vi "Alpha Ver 1.1.vi"() -> ()   [LabVIEW 2015]
uses:
  <instrlib>/Keithley 622x LV 2009/Configure/Source/Typedefs/KE622x -- Current Range.ctl
  <instrlib>/Keithley 622x LV 2009/Configure/Source/Typedefs/KE622x -- Current Ranges.ctl
  <instrlib>/Keithley 622x LV 2009/Typedefs/KE622x -- On Off Control.ctl
  <instrlib>/Keithley 622x LV 2009/Utility/Typedefs/KE622x -- Instrument Type.ctl
  <instrlib>/Keithley 622x LV 2009/Configure/Source/Typedefs/KE622x -- Voltage Limit.ctl
  <instrlib>/Keithley 2000/Public/Configure/Configure DC Volts.vi
  <userlib>/LV-Link3/PolySubVIs/DtCreateAinChan.vi
  <userlib>/LV-Link3/PolySubVIs/DtOLReadMultipleSingle.vi
  <instrlib>/Keithley 2000/Keithley 2000.lvlib
  <instrlib>/Keithley 622x LV 2009/Keithley 622x.lvlib
panel:
  out "DAQ A4":dbl format="%#_13g"
  out "DAQ_clust":T1
  out "DAQ A3":dbl format="%#_13g"
  out "DAQ A2":dbl format="%#_13g"
  out "DAQ A1":dbl format="%#_13g"
  out "Real stop cur":dbl format="%#_13g"
  out "Real start cur":dbl format="%#_13g"
  in  "Stop cur prefix":u16(ring)=2
  in  "Start cur prefix":u16(ring)=2
  out "MULTIPLE GRAPHS":cluster{dbl[], dbl[]}[](graph)
  in  "X-Axis":T2(ring)
  in  "Range":u8(ring)=20 items=["100nV", "200nV", "500nV", "1µV", "2µV", "5µV", "10µV", "20µV", "50µV", "100µV", "200µV", "500µV", "1mV", "2mV", "5mV", "10mV", "20mV", "50mV", "100mV", "200mV", "500mV", "1V"]
  in  "Display Type copy":u16(ring)=3 items=["X %", "Y %", "X Calibrated", "Y Calibrated", "Mag %", "Mag Calibrated", "Phase Degrees", "Ratio", "ADC 1", "ADC 2", "ADC 3", "ADC 4 ", "Noise %", "Noise Calibrated", "Ref Frequency", "", ""]
  out "Units copy":string
  out "Display copy":dbl format="%.3f"
  out "Overload":bool
  out "Display":dbl format="%.3f"
  out "Units":string
  in  "Display Type":u16(ring)=2 items=["X %", "Y %", "X Calibrated", "Y Calibrated", "Mag %", "Mag Calibrated", "Phase Degrees", "Ratio", "ADC 1", "ADC 2", "ADC 3", "ADC 4 ", "Noise %", "Noise Calibrated", "Ref Frequency", "", ""]
  in  "Time Constant":u16(ring) items=["MIN", "1ms", "3ms", "10ms", "30ms", "100ms", "300ms", "1s", "3s", "10s", "30s", "100s", "300s"]
  in  "Slope":u8(ring) items=["6db/octave", "12dB/octave"]
  in  "Dynamic Reserve":u16(ring) items=["High Stability", "Normal", "High Reserve"]
  in  "Auto Sensitivity":bool
  in  "Auto Measure":bool
  out "6221_error_out":errorcluster
  out "2000_error_out":errorcluster
  out "5110_error_out":errorcluster
  out "Input Mode":i32(ring) items=[" Voltage Input (A or A-B) ", "Current Input 10E6 V/A", "Current Input 10E8 V/A"]
  out "5110":refnum<visa-resource-name>
  in  "GPIB Address":i8=11 min=1 max=32 step=1
  out "DAQ A0":dbl format="%#_13g"
  out "2000":dbl format="%#_13g"
  in  "Device":string(combo)
  in  "Number \nof points":i32
  in  "Folder\nprename":string
  out "TIME GRAPH":cluster{dbl[], dbl[]}[](graph)
  out "T0":u32
  out "LIMIT":bool
  out "LIMIT":bool
  out "Error Code":string
  in  "Comments":string
  out "file":refnum<file>
  out "2000":refnum<visa-resource-name>
  out "6221":refnum<visa-resource-name>
  out "Step  (A)":dbl=5e-05 format="%#_3p"
  in  "Stop\ncurrent (A)":dbl=2.0 format="%#_6p"
  in  "Start \ncurrent (A)":dbl=1.0 format="%#_6p"
  in  "Check For SCPI Errors? (T)":bool=TRUE
  out "Interlock Tripped?":bool
  out "Compliance?":bool
  in  "Turn Off Output \nIf Compliance?":bool=TRUE
  in  "Turning ON/OFF\ncurrent output":T3=enum."On"
  in  "Range Selection":T4={"Auto Range?"=TRUE, "Man / Selected\nRange"=enum."2nA"}
  # "FILE CONFIGURATION"
  # "ADMIN PANEL"
  # "KEITHLEY 6221 CONFIGURATION (ADMIN ONLY)"
  # "KEITHLEY DAQ CONFIGURATION (ADMIN ONLY)"
  # "PRINCETON LOCK-IN AMP (ADMIN ONLY)"
  # "I don't know what the hell it is,\njust don't touch it"
  # "SENSITIVITY"
  # "INPUT CONFIGURATION"
  # "READINGS"
  # "START, STOP, STEP, CONFIGURATION"
  # "IF ON"
  # "Output Channels Time - Constant \nSlope & Dynamic Reserve"
  # "Compliance = Limiting output voltage\nThis switch determines if we want to switch \noff the current output if wee exceed compliance"
  # "LOCK-IN READINGS"
  # "RIGHT DISPLAY"
  # "LEFT DISPLAY"
  # "There is a safe switch at \nthe back of the instrument \nThis indicator shows if it is on"
  # "You have hit a damn jackpot \nby exceeding the limited voltage\nCongrats"
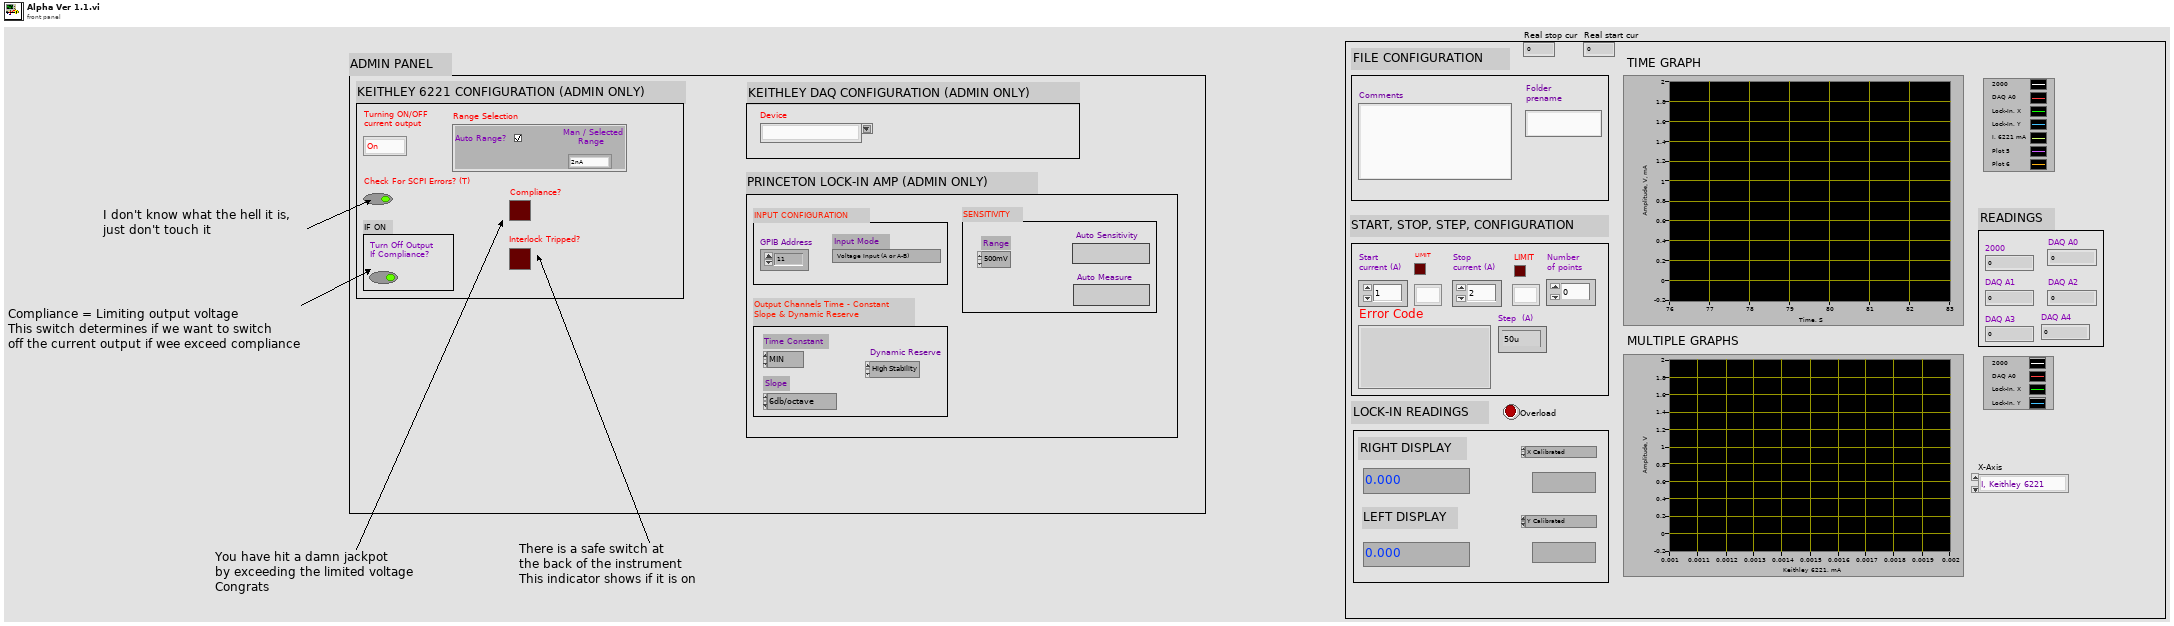
[diagram p1: front panel]
types:
  T1 = cluster{"Task out":i32, "Actual Number of Channels":u32, "error out":errorcluster}
  T2 = enum16{"I, Keithley 6221", "V, Keithley 2000", "V, Keithley DAQ A0", "V, Keithley DAQ A1", "V, Keithley DAQ A2", "V, Keithley DAQ A3", "V, Lock-In X", "V, Lock-In Y"}
  T3 = typedef "Keithley 622x.lvlib/KE622x -- On Off Control.ctl" = enum16{"Off", "On"}
  T4 = typedef "Keithley 622x.lvlib/KE622x -- Current Range.ctl" = cluster{"Auto Range?":bool, "Man / Selected\nRange":T5}
  T5 = typedef "Keithley 622x.lvlib/KE622x -- Current Ranges.ctl" = enum16{"2nA", "20nA", "200nA", "2uA", "20uA", "200uA", "2mA", "20mA", "100mA"}
  T6 = typedef "Keithley 622x.lvlib/KE622x -- Instrument Type.ctl" = enum16{"KE6220", "KE6221"}
  T7 = typedef "Keithley 622x.lvlib/KE622x -- Voltage Limit.ctl" = dbl
  T8 = cluster{"Task out":i32, "error out":errorcluster}
  T9 = cluster{dbl[], dbl[], dbl[], dbl[], dbl[], dbl[], dbl[], dbl[], dbl[]}
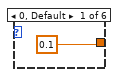
[diagram p2: hidden frame]
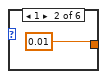
[diagram p3: hidden frame]
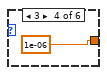
[diagram p4: hidden frame]
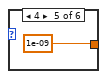
[diagram p5: hidden frame]
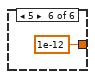
[diagram p6: hidden frame]
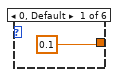
[diagram p7: hidden frame]
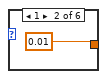
[diagram p8: hidden frame]
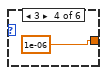
[diagram p9: hidden frame]
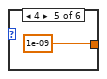
[diagram p10: hidden frame]
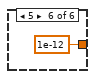
[diagram p11: hidden frame]
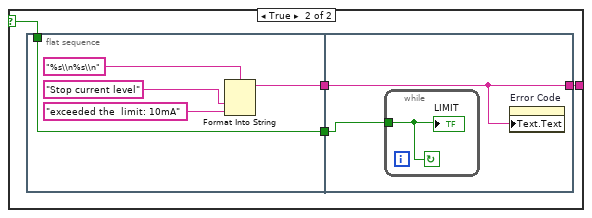
[diagram p12: hidden frame]
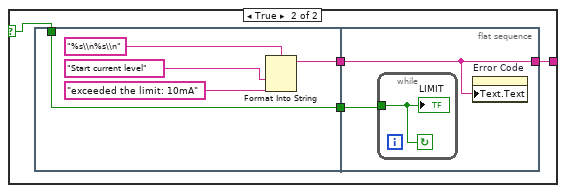
[diagram p13: hidden frame]
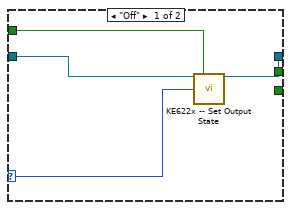
[diagram p14: hidden frame]
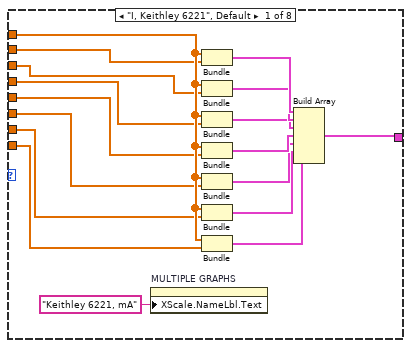
[diagram p15: hidden frame]
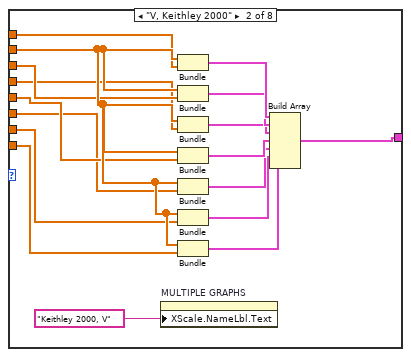
[diagram p16: hidden frame]
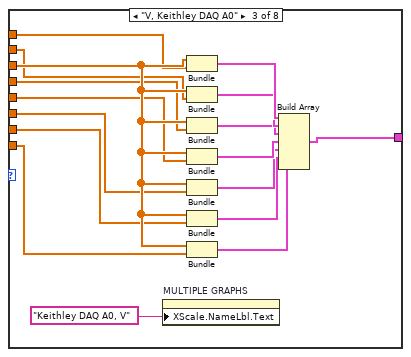
[diagram p17: hidden frame]
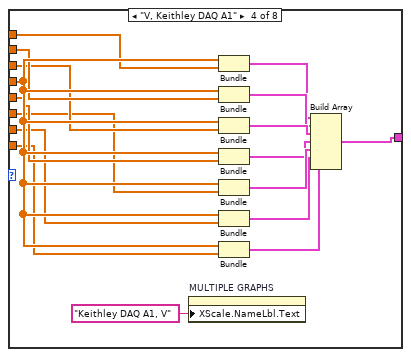
[diagram p18: hidden frame]
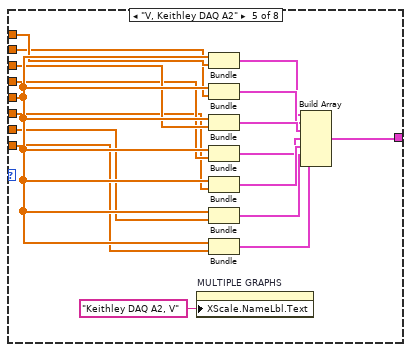
[diagram p19: hidden frame]
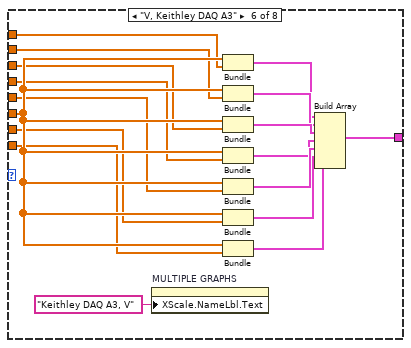
[diagram p20: hidden frame]
diagram:
  n1 = flat-sequence {
    tunnel: [w173] -> w7
    tunnel: [w172] -> w6
    tunnel: [w171] -> w5
    tunnel: [w170] -> w4
    tunnel: [w169] -> w3
    tunnel: [w168] -> w2
    tunnel: [w157] -> w1
    tunnel: w7 -> [w755]
    tunnel: w6 -> [w754]
    tunnel: w5 -> [w753]
    tunnel: w4 -> [w752]
    tunnel: w3 -> [w751]
    tunnel: w2 -> [w750]
    tunnel: w1 -> [w749]
    frame #0 {
      # "File configuration"
      # "Start, Stop, Step"
      # "Time Intit"
      # "Initializing instruments"
      n2 = flat-sequence {
        frame #0 {
          w16 = TRUE  # reset
          w15 = FALSE  # ID query
          # "Initialize Lock-In 5110"
          # "Initialize Keithley 2000"
          # "Initialize Keithley 6221"
          n3 = call <instrlib>:"Initialize.vi"("VISA resource name"=refnum<visa-resource-name> "KEITHLEY_MULTIMETER") -> ("VISA resource name out"=w20:refnum<visa-resource-name>)  [unwired: 17 in, 1 out]
          n4 = call <instrlib>:"Initialize.vi"("VISA resource name"=refnum<visa-resource-name> "KEITHLEY_DC_AC_CURRENT_SOURCE", "Error Queue Option"=enum16{"Clear Error Queue", "Error Query"}."Clear Error Queue", "Instrument Type"=KE622x_--_Instrument_Type."KE6221") -> ("VISA resource name out"=→"6221":refnum<visa-resource-name>, "error out"=→"6221_error_out":errorcluster)  [unwired: 11 in]
          n5 = call "SR51XX Initialize"("VISA session (for class)"=refnum<visa-resource-name> "LOCK_IN_5110_PRINCETON", "Interface"=FALSE, "ID query"=w15, "GPIB Address"="GPIB Address", "reset"=w16) -> ("VISA session"=→"5110":refnum<visa-resource-name>, "error out"=→"5110_error_out":errorcluster)  [unwired: 8 in, 1 out]
          n6 = call-poly <instrlib>:"Configure Measurement.vi"("VISA resource name"=w20) -> ("VISA resource name out"=→"2000":refnum<visa-resource-name>, "error out"=→"2000_error_out":errorcluster)  [unwired: 17 in]
        }
        frame #1 {
          # "Initialize Keithley DAQ \n(getting board name)"
          n7 = call <userlib>:"DtOLGetBoardNames.vi"() -> ("Number of boards"=w25:u32)  [unwired: 9 in, 2 out]
          n8 = Initialize Array("", w25) -> (w27:string[])
          n9 = for {
            N: w25 -> [_]
            shift-right: [w33] -> w30
            shift-left: w27 -> [w34]
            i -> [w32]
            n10 = Add(x=1, y=w32) -> (x+y=w36:i32)
            n11 = call <userlib>:"DtOLGetBoardNames.vi"("Select Board"=w36) -> ("Board Name"=w31:string)  [unwired: 8 in, 2 out]
            n12 = Replace Array Subset(array=w34, new element=w31, index=w32) -> (w33:string[])
          }
          n13 = Index Array(array=w30, index=0) -> (element=w29:string)
          n14 = property on="Device" class="CmbBox"("Strings[]"=w30, "Value"=w29) -> ()  [unwired: 2 in, 2 out]
        }
        frame #2 {
          # "Calculating steps by number\nof points"
          # "Putting in a loop \ninstead of \"STOP\""
          n15 = local read "Real stop cur"() -> (w53:dbl)
          n16 = local read "Real start cur"() -> (w54:dbl)
          n17 = case shown="2" "Start cur prefix" {
            tunnel: [0.1 0.01 0.001 1e-06 1e-09 1e-12] -> w42
            frame 0, Default {
            }
            frame 1 {
            }
            frame 2 {
            }
            frame 3 {
            }
            frame 4 {
            }
            frame 5 {
            }
          }
          n18 = case shown="2" "Stop cur prefix" {
            tunnel: [0.1 0.01 0.001 1e-06 1e-09 1e-12] -> w40
            frame 0, Default {
            }
            frame 1 {
            }
            frame 2 {
            }
            frame 3 {
            }
            frame 4 {
            }
            frame 5 {
            }
          }
          n19 = Subtract(x=w53, y=w54) -> (x-y=w56:dbl)
          n20 = Multiply(x=w42, y="Start \ncurrent (A)") -> (x*y=w38:dbl)
          "Real start cur" <- w38
          n21 = Divide(x=w56, y="Number \nof points") -> (x/y=→"Step  (A)":dbl)
          n22 = Multiply(x=w40, y="Stop\ncurrent (A)") -> (x*y=w37:dbl)
          "Real stop cur" <- w37
          n23 = Greater?(x=w37, y=T7 0.01) -> (0:w48:bool)
          n24 = Greater?(x=w38, y=T7 0.01) -> (0:w47:bool)
          n25 = case shown="False" w48 {
            selector: w48 -> [_ w72]
            tunnel: [w69 w75] -> w50
            frame False {
              n26 = Format Into String(format string="%s\\n", "Start current level is OK" ("false string")) -> (resulting string=w69:string)  [unwired: 2 in, 1 out]
            }
            frame True {
              n27 = flat-sequence {
                tunnel: [w77] -> w74
                tunnel: [w76] -> w73
                tunnel: w72 -> [w76]
                tunnel: [w81] -> w75
                tunnel: w74 -> [w81]
                tunnel: w73 -> [w82]
                frame #0 {
                  n28 = Format Into String(format string="%s\\n%s\\n", "Stop current level" ("String"), "exceeded the  limit: 10mA" ("input 2")) -> (resulting string=w77:string)  [unwired: 2 in, 1 out]
                }
                frame #1 {
                  n29 = while {
                    tunnel: w82 -> [w83]
                    stop <- w83 continue-if-true
                    "LIMIT" <- w83
                  }
                  n30 = property on="Error Code" class="Str"("Text.Text"=w81) -> ()  [unwired: 2 in, 2 out]
                }
              }
            }
          }
          n31 = case shown="False" w47 {
            selector: w47 -> [_ w88]
            tunnel: [w84 w90] -> w49
            frame False {
              n32 = Format Into String(format string="%s\\n", "Start current level is OK" ("false string")) -> (resulting string=w84:string)  [unwired: 2 in, 1 out]
            }
            frame True {
              n33 = flat-sequence {
                tunnel: [w92] -> w89
                tunnel: w88 -> [w91]
                tunnel: [w91] -> w87
                tunnel: [w96] -> w90
                tunnel: w89 -> [w96]
                tunnel: w87 -> [w97]
                frame #0 {
                  n34 = Format Into String(format string="%s\\n%s\\n", "Start current level" ("String"), "exceeded the limit: 10mA" ("input 2")) -> (resulting string=w92:string)  [unwired: 2 in, 1 out]
                }
                frame #1 {
                  n35 = while {
                    tunnel: w97 -> [w98]
                    stop <- w98 continue-if-true
                    "LIMIT" <- w98
                  }
                  n36 = property on="Error Code" class="Str"("Text.Text"=w96) -> ()  [unwired: 2 in, 2 out]
                }
              }
            }
          }
          n37 = Concatenate Strings(w49, w50) -> (→"Error Code":string)
        }
        frame #3 {
          n38 = flat-sequence {
            frame #0 {
              # "Creating folder&file"
              n39 = call "folder_creation.vi"("Name"="Folder\nprename") -> ("String"=w100:string)
              n40 = call "file_creation.vi"("String"=w100) -> ("refnum out"=→"file":refnum<file>)
            }
            frame #1 {
              # "Creating comments"
              n41 = local read "file"() -> (w102:refnum<file>)
              n42 = Format Into String(format string="# %s\\n", initial string=w102, "Comments") -> ()  [unwired: 1 in, 2 out]
            }
            frame #2 {
              # "Writing instr params"
              n43 = local read "5110"() -> (w110:refnum<visa-resource-name>)
              n44 = local read "Real stop cur"() -> (w108:dbl)
              n45 = local read "file"() -> (w105:refnum<file>)
              n46 = local read "Real start cur"() -> (w109:dbl)
              n47 = call "com_inst.vi"("Stop current"=w108, "Start current"=w109, "VISA session (for class)"=w110) -> ("concatenated string"=w106:string)
              n48 = Format Into String(format string="# %s\\n", initial string=w105, w106) -> ()  [unwired: 1 in, 2 out]
            }
            frame #3 {
              # "Adding headlines"
              n49 = local read "file"() -> (w121:refnum<file>)
              n50 = Format Into String(format string="# %-6s  %-12s %-12s %-12s %-12s %-12s  %-12s %-14s %-14s\\n", initial string=w121, "t, ms" ("input 3"), "2000, V" ("input 1"), "DAQ A0" ("input 2"), "DAQ A1" ("input 2"), "DAQ A2" ("input 2"), "DAQ A3" ("input 2"), "5110_X" ("input 3"), "5110_Y " ("input 3"), "6221, mA" ("input 3")) -> ()  [unwired: 1 in, 2 out]
            }
          }
        }
      }
      n51 = Tick Count (ms)() -> (millisecond timer value=→"T0":u32)
    }
    frame #1 {
      # "Configuring Keithley DAQ just before measuments"
      # "Configuring Keithley 6221 just before measuments"
      n52 = flat-sequence {
        tunnel: [w132] -> w122
        tunnel: [w150] -> _
        tunnel: [w152] -> _
        tunnel: w122 -> [w151]
        frame #0 {
          # "Current range \nselection check"
          # "Checking for compliance\nand interlock errors"
          n53 = local read "6221"() -> (w135:refnum<visa-resource-name>)
          n54 = call <instrlib>:"KE622x -- Set Current Range.vi"("Resource In"=w135, "Current Range In"="Range Selection", "Read Back Set Values? (T)"=FALSE) -> ("Resource Out (dupl)"=w140:refnum<visa-resource-name>)  [unwired: 10 in, 2 out]
          n55 = case shown="\"On\"" "Turning ON/OFF\ncurrent output" {
            selector: "Turning ON/OFF\ncurrent output" -> [w144 _]
            tunnel: [_ w148] -> w138
            tunnel: [_ w147] -> w139
            tunnel: "Check For SCPI Errors? (T)" -> [w143 _]
            tunnel: w140 -> [w141 w146]
            tunnel: [w142 w145] -> w132
            frame "Off" {
              n56 = call <instrlib>:"KE622x -- Set Output State.vi"("Resource In"=w141, "Check For SCPI Errors? (T)"=w143, "Output State"=w144) -> ("Resource Out (dupl)"=w142:refnum<visa-resource-name>)  [unwired: 11 in, 1 out]
            }
            frame "On" {
              n57 = call <instrlib>:"KE622x -- Turn Output On And Check For Errors.vi"("Resource In"=w146, "Turn Off Output If Compliance?"="Turn Off Output \nIf Compliance?") -> ("Resource Out (dupl)"=w145:refnum<visa-resource-name>, "Interlock Tripped?"=w148:bool, "Compliance?"=w147:bool)  [unwired: 10 in, 1 out]
            }
          }
          "Interlock Tripped?" <- w138
          "Compliance?" <- w139
        }
        frame #1 {
          # "Setting start current"
          n58 = local read "Real start cur"() -> (w150:dbl)
          n59 = Wait (ms)(milliseconds to wait=u32 100) -> ()  [unwired: 1 out]
          n60 = call <instrlib>:"KE622x -- Set Current Level.vi"("Resource In"=w151, "Current Level (A) In"=w150) -> ("Resource Out (dupl)"=w152:refnum<visa-resource-name>)  [unwired: 12 in, 1 out]
        }
      }
      n61 = flat-sequence {
        frame #0 {
          w127 = 100 items=["SingleEnded"=100, "Differential"=101] ("Channel Type")
          # "Configure the input channel"
          n62 = call-poly <userlib>:"DtOLCreateTask.vi"("Channel Type"=w127, "Range Min"=-10.0, "Range Max"=10.0, "Board Name"="Device", "Channel"="0:4" ("Channels")) -> ("Task out"=w126:i32, "Actual Number of Channels"=w125:u32, "error out"=w124:errorcluster)  [unwired: 8 in]
          n63 = Bundle("Task out"=w126, "Actual Number of Channels"=w125, "error out"=w124) -> (→"DAQ_clust":T1)  [unwired: 1 in]
        }
      }
    }
    frame #2 {
      n64 = local read "5110"() -> (w164:refnum<visa-resource-name>)
      n65 = local read "2000"() -> (w163:refnum<visa-resource-name>)
      n66 = local read "6221"() -> (w162:refnum<visa-resource-name>)
      n67 = local read "5110_error_out"() -> (w161:errorcluster)
      n68 = local read "6221_error_out"() -> (w160:errorcluster)
      n69 = local read "2000_error_out"() -> (w159:errorcluster)
      n70 = local read "DAQ_clust"() -> (w158:T1)
      n71 = while {
        shift-right: [w239] -> _
        shift-left: dbl[] [] -> [w396]
        shift-right: [w240] -> _
        shift-left: i32[] [] -> [w395]
        tunnel: w163 -> [w393]
        tunnel: w162 -> [w392]
        shift-right: [w235] -> _
        shift-left: dbl[] [] -> [w385]
        tunnel: [w384] -> w173
        tunnel: [w383] -> w172
        tunnel: [w381] -> w171
        tunnel: [w378] -> w170
        tunnel: w164 -> [w375]
        tunnel: w161 -> [w374]
        tunnel: w160 -> [w366]
        tunnel: w159 -> [w365]
        tunnel: [w316] -> w169
        tunnel: [w313] -> w168
        shift-right: [w234] -> _
        shift-left: dbl[] [] -> [w312]
        shift-right: [w233] -> _
        shift-left: dbl[] [] -> [w311]
        shift-right: [w241] -> _
        shift-left: dbl[] [] -> [w308]
        tunnel: w158 -> [w265]
        tunnel: [w264] -> w157
        shift-right: [w238] -> _
        shift-left: dbl[] [] -> [w263]
        shift-right: [w237] -> _
        shift-left: dbl[] [] -> [w262]
        shift-right: [w236] -> _
        shift-left: dbl[] [] -> [w261]
        i -> [w367]
        stop <- w386 stop-if-true
        # "V, DAQ A3"
        # "V, DAQ A2"
        # "V, DAQ A1"
        # "Y-V, 5110"
        # "X-V, 5110"
        # "I, 6221"
        # "Config delay"
        # "Control subVI 5110"
        # "Read config 5110"
        # "Measurement config 5110"
        # "Time config 5110"
        # "Configuring Right Display 5110"
        # "Configuring Left Display 5110"
        # "Setting 6221 current"
        # "Delay before measuremens"
        # "Getting the data from DAQ and 2000"
        # "Changing input current"
        # "Time"
        # "V, DAQ A0"
        # "V, 2000"
        n72 = local read "T0"() -> (w394:u32)
        n73 = Quotient & Remainder(x=w367, y=10) -> (floor(x/y)=w372:i32)  [unwired: 1 out]
        n74 = Equal?(x=0, y=w367) -> (x = y?=w369:bool)
        n75 = Subtract(x=w356, y=w394) -> (x-y=w276:u32)
        n76 = Equal?(x=1, y=w372) -> (x = y?=w368:bool)
        n77 = flat-sequence {
          tunnel: w393 -> [w543]
          tunnel: [w543] -> w307
          tunnel: w392 -> [w542]
          tunnel: [w542] -> w305
          tunnel: w375 -> [w540]
          tunnel: [w540] -> w303
          tunnel: [w539] -> w301
          tunnel: w374 -> [w539]
          tunnel: w369 -> [w538]
          tunnel: [w538] -> w299
          tunnel: w368 -> [w537]
          tunnel: [w537] -> w297
          tunnel: w366 -> [w536]
          tunnel: [w536] -> w295
          tunnel: w365 -> [w535]
          tunnel: [w535] -> w293
          tunnel: [w534] -> w356
          tunnel: [w533] -> w266
          tunnel: w265 -> [w533]
          tunnel: w307 -> [w558]
          tunnel: [w558] -> w306
          tunnel: w305 -> [w557]
          tunnel: [w557] -> w304
          tunnel: w303 -> [w556]
          tunnel: [w556] -> w302
          tunnel: w301 -> [w555]
          tunnel: [w555] -> w300
          tunnel: w299 -> [w554]
          tunnel: [w554] -> w298
          tunnel: w297 -> [w553]
          tunnel: [w553] -> w296
          tunnel: w295 -> [w552]
          tunnel: [w552] -> w294
          tunnel: w293 -> [w551]
          tunnel: [w551] -> w292
          tunnel: [w544] -> w267
          tunnel: w266 -> [w544]
          tunnel: w306 -> [w571]
          tunnel: [w571] -> w355
          tunnel: w304 -> [w570]
          tunnel: [w570] -> w354
          tunnel: w302 -> [w569]
          tunnel: w300 -> [w566]
          tunnel: [w565] -> w353
          tunnel: [w564] -> w352
          tunnel: w298 -> [w563]
          tunnel: [w563] -> w351
          tunnel: w296 -> [w562]
          tunnel: w294 -> [w561]
          tunnel: [w561] -> w350
          tunnel: w292 -> [w560]
          tunnel: [w560] -> w349
          tunnel: [w559] -> w268
          tunnel: w267 -> [w559]
          tunnel: w355 -> [w596]
          tunnel: [w596] -> w348
          tunnel: w354 -> [w595]
          tunnel: [w595] -> w347
          tunnel: w353 -> [w592]
          tunnel: [w591] -> w346
          tunnel: w352 -> [w590]
          tunnel: [w589] -> w345
          tunnel: w351 -> [w587]
          tunnel: [w587] -> w344
          tunnel: w350 -> [w594]
          tunnel: [w594] -> w343
          tunnel: w349 -> [w593]
          tunnel: [w593] -> w342
          tunnel: ["Auto Measure"] -> w341
          tunnel: ["Auto Sensitivity"] -> w340
          tunnel: [w582] -> w339
          tunnel: [w579] -> w269
          tunnel: w268 -> [w579]
          tunnel: w348 -> [w615]
          tunnel: [w615] -> w291
          tunnel: w347 -> [w614]
          tunnel: [w614] -> w290
          tunnel: w346 -> [w607]
          tunnel: w345 -> [w605]
          tunnel: [w604] -> w289
          tunnel: w344 -> [w611]
          tunnel: [w611] -> w288
          tunnel: w343 -> [w613]
          tunnel: [w613] -> w287
          tunnel: w342 -> [w612]
          tunnel: [w612] -> w286
          tunnel: w341 -> [w609]
          tunnel: [w609] -> w285
          tunnel: w340 -> [w610]
          tunnel: [w610] -> w284
          tunnel: w339 -> [w600]
          tunnel: [w600] -> w283
          tunnel: [w606] -> w282
          tunnel: ["Time Constant"] -> w281
          tunnel: ["Slope"] -> w280
          tunnel: [w597] -> w270
          tunnel: w269 -> [w597]
          tunnel: [w639] -> w338
          tunnel: [w638] -> w337
          tunnel: [w624] -> w336
          tunnel: [w637] -> w335
          tunnel: [w636] -> w334
          tunnel: [w635] -> w333
          tunnel: [w634] -> w332
          tunnel: [w633] -> w331
          tunnel: [w626] -> w330
          tunnel: [w629] -> w329
          tunnel: [w627] -> w328
          tunnel: [w632] -> w327
          tunnel: [w617] -> w256
          tunnel: w280 -> [w632]
          tunnel: w281 -> [w627]
          tunnel: w282 -> [w630]
          tunnel: w283 -> [w626]
          tunnel: w284 -> [w633]
          tunnel: w285 -> [w634]
          tunnel: w286 -> [w635]
          tunnel: w287 -> [w636]
          tunnel: w288 -> [w637]
          tunnel: w289 -> [w625]
          tunnel: w290 -> [w638]
          tunnel: w291 -> [w639]
          tunnel: [w616] -> w271
          tunnel: w270 -> [w616]
          tunnel: w338 -> [w663]
          tunnel: [w663] -> w326
          tunnel: w337 -> [w662]
          tunnel: [w662] -> w325
          tunnel: w336 -> [w649]
          tunnel: w335 -> [w661]
          tunnel: [w661] -> w324
          tunnel: w334 -> [w660]
          tunnel: [w660] -> w323
          tunnel: w333 -> [w659]
          tunnel: [w659] -> w322
          tunnel: w332 -> [w658]
          tunnel: [w658] -> w321
          tunnel: w331 -> [w657]
          tunnel: [w657] -> w320
          tunnel: w330 -> [w650]
          tunnel: w329 -> [w647]
          tunnel: [w646] -> w319
          tunnel: w328 -> [w651]
          tunnel: w327 -> [w652]
          tunnel: [w648] -> w318
          tunnel: [w645] -> w317
          tunnel: [w641] -> w255
          tunnel: [w640] -> w272
          tunnel: w271 -> [w640]
          tunnel: [w667] -> w390
          tunnel: w367 -> [w675]
          tunnel: [w671] -> w386
          tunnel: [w665] -> w388
          tunnel: [w673] -> w387
          tunnel: [w670] -> w364
          tunnel: [w669] -> w363
          tunnel: [w668] -> w362
          tunnel: [w666] -> w361
          tunnel: [w665] -> w257
          tunnel: w317 -> [_]
          tunnel: w318 -> [w668]
          tunnel: w319 -> [w666]
          tunnel: w320 -> [_]
          tunnel: w321 -> [_]
          tunnel: w322 -> [w670]
          tunnel: w323 -> [w669]
          tunnel: w324 -> [_]
          tunnel: w325 -> [w673]
          tunnel: w326 -> [w667]
          tunnel: [w664] -> w273
          tunnel: w272 -> [w664]
          tunnel: w390 -> [w687]
          tunnel: [w687] -> w389
          tunnel: w388 -> [w686]
          tunnel: w387 -> [w685]
          tunnel: [w684] -> w382
          tunnel: [w683] -> w379
          tunnel: w364 -> [w681]
          tunnel: w363 -> [w682]
          tunnel: w362 -> [w679]
          tunnel: w361 -> [w680]
          tunnel: [w681] -> w360
          tunnel: [w680] -> w357
          tunnel: [w679] -> w314
          tunnel: [w678] -> w274
          tunnel: w273 -> [w678]
          tunnel: w389 -> [w695]
          tunnel: [w695] -> w391
          tunnel: w382 -> [w693]
          tunnel: [w693] -> w380
          tunnel: w379 -> [w692]
          tunnel: [w692] -> w377
          tunnel: w360 -> [w691]
          tunnel: [w691] -> w359
          tunnel: [w690] -> w358
          tunnel: w357 -> [w690]
          tunnel: [w689] -> w315
          tunnel: w314 -> [w689]
          tunnel: [w688] -> w275
          tunnel: w274 -> [w688]
          tunnel: [w732] -> w201
          tunnel: [w699] -> w200
          tunnel: [w731] -> w199
          tunnel: [w730] -> w198
          tunnel: [w729] -> w197
          tunnel: [w728] -> w196
          tunnel: [w700] -> w195
          tunnel: [w732] -> w194
          tunnel: [w727] -> w193
          tunnel: [w726] -> w192
          tunnel: [w725] -> w191
          tunnel: w275 -> [w722]
          tunnel: w315 -> [w726]
          tunnel: w358 -> [w727]
          tunnel: w359 -> [w723]
          tunnel: w377 -> [w728]
          tunnel: w380 -> [w729]
          tunnel: w391 -> [w724]
          tunnel: [w698] -> w190
          tunnel: [w697] -> w189
          tunnel: [w696] -> w188
          tunnel: [w736] -> w264
          tunnel: [w737] -> w313
          tunnel: [w738] -> w316
          tunnel: [w739] -> w376
          tunnel: [w740] -> w186
          tunnel: [w741] -> w378
          tunnel: [w742] -> w381
          tunnel: [w743] -> w383
          tunnel: [w744] -> w384
          tunnel: [w745] -> w185
          tunnel: [w746] -> w260
          tunnel: w201 -> [w746]
          tunnel: w200 -> [w745]
          tunnel: w199 -> [w744]
          tunnel: w198 -> [w743]
          tunnel: w197 -> [w742]
          tunnel: w196 -> [w741]
          tunnel: w195 -> [w740]
          tunnel: w194 -> [w739]
          tunnel: w193 -> [w738]
          tunnel: w192 -> [w737]
          tunnel: w191 -> [w736]
          tunnel: [w735] -> w184
          tunnel: w190 -> [w735]
          tunnel: [w734] -> w183
          tunnel: w189 -> [w734]
          tunnel: w188 -> [w733]
          tunnel: [w733] -> w187
          frame #0 {
            n78 = Wait Until Next ms Multiple(millisecond multiple=u32 500) -> (millisecond timer value=w534:u32)
          }
          frame #1 {
            n79 = control-ref of="Range"() -> (w550:refnum<vi>)
            n80 = control-ref of="Auto Sensitivity"() -> (w549:refnum<vi>)
            n81 = control-ref of="Auto Measure"() -> (w548:refnum<vi>)
            n82 = control-ref of="Time Constant"() -> (w545:refnum<vi>)
            n83 = control-ref of="Slope"() -> (w546:refnum<vi>)
            n84 = control-ref of="Dynamic Reserve"() -> (w547:refnum<vi>)
            n85 = call "cont_ver_1.0.vi"("Dynamic Reserve"=w547, "Slope"=w546, "Time Constant"=w545, "Auto Measure"=w548, "Auto Sensitivity"=w549, "Range"=w550) -> ()
          }
          frame #2 {
            n86 = case shown="False" w562 {
              tunnel: w569 -> [w573 w578]
              tunnel: [w572 w576] -> w568
              tunnel: [w573 w575] -> w567
              tunnel: w566 -> [w572 w574]
              frame False {
              }
              frame True {
                n87 = call "SR51XX Read Preamp Input Mode"("VISA session (for class)"=w578, "error in (no error)"=w574) -> ("VISA session"=w575:refnum<visa-resource-name>, "Input Mode"=w577:i32, "error out"=w576:errorcluster)  [unwired: 15 in]
                n88 = local write "Input Mode"(w577) -> ()
              }
            }
            n89 = call "SR51XX Configure Signal Channel Input"("VISA session (for class)"=w567, "error in (no error)"=w568, "Update"=w563) -> ("VISA session"=w565:refnum<visa-resource-name>, "error out"=w564:errorcluster)  [unwired: 15 in]
          }
          frame #3 {
            n90 = local read "Input Mode"() -> (w588:i32)
            n91 = call "SR51XX Configure Sensitivity"("VISA session (for class)"=w592, "Input Mode"=w588, "Range"="Range", "error in (no error)"=w590, "Auto Sensitivity"="Auto Sensitivity", "Auto Measure"="Auto Measure", "Update"=w587) -> ("Range Annotations Out[]"=w580:string[], "VISA session"=w591:refnum<visa-resource-name>, "Auto Sensitivity out"=w584:bool, "Auto Measure out"=w583:bool, "Range Out"=w582:u8, "error out"=w589:errorcluster)  [unwired: 7 in]
            n92 = property on="Range" class="Ring (strict)"("Strings []"=w580) -> ()  [unwired: 2 in, 2 out]
            n93 = local write "Auto Sensitivity"(w584) -> ()
            n94 = local write "Auto Measure"(w583) -> ()
            n95 = local write "Range"(w582) -> ()
          }
          frame #4 {
            n96 = Or(x=w610, y=w609) -> (x .or. y?=w608:bool)
            n97 = call "SR51XX Configure Output Channels - Slope, TC and Dyn Reserve"("VISA session (for class)"=w607, "Time Constant"="Time Constant", "Slope"="Slope", "Check TC"=w608, "Dynamic Reserve"="Dynamic Reserve", "error in (no error)"=w605, "Range"=w600, "Update"=w611) -> ("VISA session"=w606:refnum<visa-resource-name>, "Slope Out"=w601:u8, "Time Constant Out"=w602:u16, "error out"=w604:errorcluster)  [unwired: 8 in]
            n98 = local write "Slope"(w601) -> ()
            n99 = local write "Time Constant"(w602) -> ()
          }
          frame #5 {
            n100 = local read "Input Mode"() -> (w631:i32)
            n101 = call "SR5110 Read Output"("VISA session (for class)"=w630, "Input Mode"=w631, "Time Constant"=w627, "Display Type"="Display Type", "Range"=w626, "error in (no error)"=w625, "Slope"=w632) -> ("Units"=w619:string, "Display Precision"=w623:i32, "Display"=w618:dbl, "VISA session"=w629:refnum<visa-resource-name>, "Available Display Types Out"=w622:string[], "Overload"=→"Overload":bool, "error out"=w624:errorcluster)  [unwired: 4 in, 2 out]
            "Units" <- w619
            "Display" <- w618
            n102 = property on="Display Type" class="Ring (strict)"("Strings []"=w622) -> ()  [unwired: 2 in, 2 out]
            n103 = property on="Display" class="DigNum (strict)"("Precision"=w623) -> ()  [unwired: 2 in, 2 out]
            n104 = call "pref_to_num.vi"("string"=w619) -> ("Numeric"=w620:dbl)
            n105 = Multiply(x=w620, y=w618) -> (x*y=w617:dbl)
          }
          frame #6 {
            n106 = local read "Input Mode"() -> (w656:i32)
            n107 = call "SR5110 Read Output"("VISA session (for class)"=w647, "Input Mode"=w656, "Time Constant"=w651, "Display Type"="Display Type copy", "Range"=w650, "error in (no error)"=w649, "Slope"=w652) -> ("Units"=w644:string, "Display Precision"=w653:i32, "Display"=w643:dbl, "VISA session"=w646:refnum<visa-resource-name>, "Reference Unlock"=w645:bool, "Available Display Types Out"=w654:string[], "error out"=w648:errorcluster)  [unwired: 4 in, 2 out]
            "Display copy" <- w643
            "Units copy" <- w644
            n108 = property on="Display Type copy" class="Ring (strict)"("Strings []"=w654) -> ()  [unwired: 2 in, 2 out]
            n109 = property on="Display copy" class="DigNum (strict)"("Precision"=w653) -> ()  [unwired: 2 in, 2 out]
            n110 = call "pref_to_num.vi"("string"=w644) -> ("Numeric"=w642:dbl)
            n111 = Multiply(x=w642, y=w643) -> (x*y=w641:dbl)
          }
          frame #7 {
            n112 = local read "Step  (A)"() -> (w676:dbl)
            n113 = local read "Real start cur"() -> (w677:dbl)
            n114 = Multiply(x=w676, y=w675) -> (x*y=w674:dbl)
            n115 = Add(x=w677, y=w674) -> (x+y=w665:dbl)
            n116 = local read "Real stop cur"() -> (w672:dbl)
            n117 = Greater Or Equal?(x=w665, y=w672) -> (x >= y?=w671:bool)
          }
          frame #8 {
            n118 = call <instrlib>:"KE622x -- Set Current Level.vi"("Resource In"=w685, "Current Level (A) In"=w686, "error in (no error)"=w682) -> ("Resource Out (dupl)"=w683:refnum<visa-resource-name>, "error out"=w684:errorcluster)  [unwired: 11 in]
          }
          frame #9 {
            n119 = Wait Until Next ms Multiple(millisecond multiple=u32 50) -> ()  [unwired: 1 out]
          }
          frame #10 {
            n120 = Unbundle(w722) -> ("Task out"=w721:i32, "Actual Number of Channels"=w719:u32, "error out"=w720:errorcluster)
            n121 = call <instrlib>:"Data Read Single.vi"("VISA resource name"=w724, "error in (no error)"=w723) -> ("VISA resource name out"=w730:refnum<visa-resource-name>, "Measurement"=w732:dbl, "error out"=w731:errorcluster)  [unwired: 13 in, 2 out]
            n122 = call-poly <userlib>:"DtOLRead.vi"("Number Chan to Read"=w719, "error in (no error)"=w720, "Task in"=w721) -> ("error out"=w717:errorcluster, "2D Data out"=w716:dbl[][], "Task out"=w718:i32)  [unwired: 4 in, 2 out]
            n123 = Index Array(array=w716, index (row) #1=0 ("index (row)"), index (row) #2=1 ("index (row)"), index (row) #3=2 ("index (row)"), index (row) #4=3 ("index (row)"), index (row) #5=4 ("index (row)")) -> (element #1=w715:dbl[], element #2=w709:dbl[], element #3=w708:dbl[], element #4=w707:dbl[], element #5=w706:dbl[])  [unwired: 5 in]
            n124 = Index Array(array=w706, index=0) -> (element=w696:dbl)
            n125 = Index Array(array=w715, index=0) -> (element=w700:dbl)
            n126 = Index Array(array=w709, index=0) -> (element=w699:dbl)
            n127 = Index Array(array=w708, index=0) -> (element=w698:dbl)
            n128 = Index Array(array=w707, index=0) -> (element=w697:dbl)
            n129 = Bundle("Task out"=w718, "error out"=w717) -> (w725:T8)  [unwired: 1 in]
          }
          frame #11 {
          }
        }
        n130 = Divide(x=w276, y=u32 1000) -> (x/y=w277:dbl)
        n131 = Build Array (concatenate)(w395, w277) -> (w249:dbl[])
        n132 = local read "file"() -> (w279:refnum<file>)
        n133 = Bundle(w257, w256, w255) -> (w254:cluster{dbl, dbl, dbl})  [unwired: 1 in]
        n134 = Unbundle(w254) -> (w253:dbl, w252:dbl, w251:dbl)
        n135 = Build Array (concatenate)(w308, w253) -> (w250:dbl[])
        n136 = Build Array (concatenate)(w312, w252) -> (w243:dbl[])
        n137 = Build Array (concatenate)(w311, w251) -> (w242:dbl[])
        n138 = Bundle(w186, w185, w184, w183, "Measurement"=w260) -> (w204:cluster{dbl, dbl, dbl, dbl, "Measurement":dbl})  [unwired: 1 in]
        n139 = Unbundle(w204) -> (w258:dbl, w182:dbl, w181:dbl, w180:dbl, "Measurement"=w259:dbl)
        n140 = Unbundle(w204) -> (w202:dbl, w179:dbl, w178:dbl, w177:dbl, "Measurement"=w203:dbl)
        n141 = Build Array (concatenate)(w396, w259) -> (w248:dbl[])
        n142 = Build Array (concatenate)(w263, w258) -> (w247:dbl[])
        n143 = Build Array (concatenate)(w262, w182) -> (w246:dbl[])
        n144 = Build Array (concatenate)(w261, w181) -> (w245:dbl[])
        n145 = Build Array (concatenate)(w385, w180) -> (w244:dbl[])
        n146 = Format Into String(format string="%08d  %8.2e %12g %14.5e %12.4e %12.4e\\n", initial string=w279, w276, w203, w202, w179, w178, w177) -> ()  [unwired: 1 in, 2 out]
        n147 = Bundle(w250, w249, w248, w247, w246, w245, w244, w243, w242) -> (w214:T9)  [unwired: 1 in]
        n148 = Unbundle(w214) -> (w224:dbl[], w232:dbl[], w231:dbl[], w230:dbl[], w229:dbl[], w228:dbl[], w227:dbl[], w226:dbl[], w225:dbl[])
        n149 = Bundle(w232, w231) -> (w223:cluster{dbl[], dbl[]})  [unwired: 1 in]
        n150 = Bundle(w232, w230) -> (w222:cluster{dbl[], dbl[]})  [unwired: 1 in]
        n151 = Bundle(w232, w229) -> (w221:cluster{dbl[], dbl[]})  [unwired: 1 in]
        n152 = Bundle(w232, w228) -> (w220:cluster{dbl[], dbl[]})  [unwired: 1 in]
        n153 = Bundle(w232, w227) -> (w219:cluster{dbl[], dbl[]})  [unwired: 1 in]
        n154 = Bundle(w232, w226) -> (w218:cluster{dbl[], dbl[]})  [unwired: 1 in]
        n155 = Bundle(w232, w225) -> (w217:cluster{dbl[], dbl[]})  [unwired: 1 in]
        n156 = Bundle(w232, w224) -> (w216:cluster{dbl[], dbl[]})  [unwired: 1 in]
        n157 = Build Array(w223, w222, w221, w220, w219, w218, w217, w216) -> (→"TIME GRAPH":cluster{dbl[], dbl[]}[])
        n158 = Unbundle(w214) -> (w213:dbl[], w212:dbl[], w211:dbl[], w210:dbl[], w209:dbl[], w208:dbl[], w207:dbl[], w206:dbl[])  [unwired: 1 out]
        n159 = case shown="\"V, Lock-In Y\"" "X-Axis" {
          tunnel: [w397 w422 w439 w448 w473 w490 w507 w524] -> w205
          tunnel: w213 -> [w412 w420 w437 w455 w471 w488 w505 w522]
          tunnel: w212 -> [w411 w421 w436 w454 w470 w487 w504 w521]
          tunnel: w211 -> [w410 w419 w438 w453 w469 w486 w503 w520]
          tunnel: w210 -> [w409 w418 w435 w456 w468 w485 w502 w519]
          tunnel: w209 -> [w408 w417 w434 w452 w472 w484 w501 w518]
          tunnel: w208 -> [w407 w416 w433 w451 w467 w489 w500 w517]
          tunnel: w207 -> [w406 w415 w432 w450 w466 w483 w506 w516]
          tunnel: w206 -> [w405 w414 w431 w449 w465 w482 w499 w523]
          frame "I, Keithley 6221", Default {
            n160 = property on="MULTIPLE GRAPHS" class="XYGraph (strict)"("XScale.NameLbl.Text"="Keithley 6221, mA" ("X Scale.Name Label.Text")) -> ()  [unwired: 2 in, 2 out]
            n161 = Bundle(w412, w411) -> (w404:cluster{dbl[], dbl[]})  [unwired: 1 in]
            n162 = Bundle(w412, w410) -> (w403:cluster{dbl[], dbl[]})  [unwired: 1 in]
            n163 = Bundle(w412, w409) -> (w402:cluster{dbl[], dbl[]})  [unwired: 1 in]
            n164 = Bundle(w412, w408) -> (w401:cluster{dbl[], dbl[]})  [unwired: 1 in]
            n165 = Bundle(w412, w407) -> (w400:cluster{dbl[], dbl[]})  [unwired: 1 in]
            n166 = Bundle(w412, w406) -> (w399:cluster{dbl[], dbl[]})  [unwired: 1 in]
            n167 = Bundle(w412, w405) -> (w398:cluster{dbl[], dbl[]})  [unwired: 1 in]
            n168 = Build Array(w404, w403, w402, w401, w400, w399, w398) -> (w397:cluster{dbl[], dbl[]}[])
          }
          frame "V, Keithley 2000" {
            n169 = property on="MULTIPLE GRAPHS" class="XYGraph (strict)"("XScale.NameLbl.Text"="Keithley 2000, V" ("X Scale.Name Label.Text")) -> ()  [unwired: 2 in, 2 out]
            n170 = Bundle(w421, w420) -> (w429:cluster{dbl[], dbl[]})  [unwired: 1 in]
            n171 = Bundle(w421, w419) -> (w428:cluster{dbl[], dbl[]})  [unwired: 1 in]
            n172 = Bundle(w421, w418) -> (w427:cluster{dbl[], dbl[]})  [unwired: 1 in]
            n173 = Bundle(w421, w417) -> (w426:cluster{dbl[], dbl[]})  [unwired: 1 in]
            n174 = Bundle(w421, w416) -> (w425:cluster{dbl[], dbl[]})  [unwired: 1 in]
            n175 = Bundle(w421, w415) -> (w424:cluster{dbl[], dbl[]})  [unwired: 1 in]
            n176 = Bundle(w421, w414) -> (w423:cluster{dbl[], dbl[]})  [unwired: 1 in]
            n177 = Build Array(w429, w428, w427, w426, w425, w424, w423) -> (w422:cluster{dbl[], dbl[]}[])
          }
          frame "V, Keithley DAQ A0" {
            n178 = property on="MULTIPLE GRAPHS" class="XYGraph (strict)"("XScale.NameLbl.Text"="Keithley DAQ A0, V" ("X Scale.Name Label.Text")) -> ()  [unwired: 2 in, 2 out]
            n179 = Bundle(w438, w437) -> (w446:cluster{dbl[], dbl[]})  [unwired: 1 in]
            n180 = Bundle(w438, w436) -> (w445:cluster{dbl[], dbl[]})  [unwired: 1 in]
            n181 = Bundle(w438, w435) -> (w444:cluster{dbl[], dbl[]})  [unwired: 1 in]
            n182 = Bundle(w438, w434) -> (w443:cluster{dbl[], dbl[]})  [unwired: 1 in]
            n183 = Bundle(w438, w433) -> (w442:cluster{dbl[], dbl[]})  [unwired: 1 in]
            n184 = Bundle(w438, w432) -> (w441:cluster{dbl[], dbl[]})  [unwired: 1 in]
            n185 = Bundle(w438, w431) -> (w440:cluster{dbl[], dbl[]})  [unwired: 1 in]
            n186 = Build Array(w446, w445, w444, w443, w442, w441, w440) -> (w439:cluster{dbl[], dbl[]}[])
          }
          frame "V, Keithley DAQ A1" {
            n187 = property on="MULTIPLE GRAPHS" class="XYGraph (strict)"("XScale.NameLbl.Text"="Keithley DAQ A1, V" ("X Scale.Name Label.Text")) -> ()  [unwired: 2 in, 2 out]
            n188 = Bundle(w456, w455) -> (w458:cluster{dbl[], dbl[]})  [unwired: 1 in]
            n189 = Bundle(w456, w454) -> (w459:cluster{dbl[], dbl[]})  [unwired: 1 in]
            n190 = Bundle(w456, w453) -> (w460:cluster{dbl[], dbl[]})  [unwired: 1 in]
            n191 = Bundle(w456, w452) -> (w461:cluster{dbl[], dbl[]})  [unwired: 1 in]
            n192 = Bundle(w456, w451) -> (w462:cluster{dbl[], dbl[]})  [unwired: 1 in]
            n193 = Bundle(w456, w450) -> (w463:cluster{dbl[], dbl[]})  [unwired: 1 in]
            n194 = Bundle(w456, w449) -> (w464:cluster{dbl[], dbl[]})  [unwired: 1 in]
            n195 = Build Array(w458, w459, w460, w461, w462, w463, w464) -> (w448:cluster{dbl[], dbl[]}[])
          }
          frame "V, Keithley DAQ A2" {
            n196 = property on="MULTIPLE GRAPHS" class="XYGraph (strict)"("XScale.NameLbl.Text"="Keithley DAQ A2, V" ("X Scale.Name Label.Text")) -> ()  [unwired: 2 in, 2 out]
            n197 = Bundle(w472, w471) -> (w474:cluster{dbl[], dbl[]})  [unwired: 1 in]
            n198 = Bundle(w472, w470) -> (w475:cluster{dbl[], dbl[]})  [unwired: 1 in]
            n199 = Bundle(w472, w469) -> (w476:cluster{dbl[], dbl[]})  [unwired: 1 in]
            n200 = Bundle(w472, w468) -> (w477:cluster{dbl[], dbl[]})  [unwired: 1 in]
            n201 = Bundle(w472, w467) -> (w478:cluster{dbl[], dbl[]})  [unwired: 1 in]
            n202 = Bundle(w472, w466) -> (w479:cluster{dbl[], dbl[]})  [unwired: 1 in]
            n203 = Bundle(w472, w465) -> (w480:cluster{dbl[], dbl[]})  [unwired: 1 in]
            n204 = Build Array(w474, w475, w476, w477, w478, w479, w480) -> (w473:cluster{dbl[], dbl[]}[])
          }
          frame "V, Keithley DAQ A3" {
            n205 = property on="MULTIPLE GRAPHS" class="XYGraph (strict)"("XScale.NameLbl.Text"="Keithley DAQ A3, V" ("X Scale.Name Label.Text")) -> ()  [unwired: 2 in, 2 out]
            n206 = Bundle(w489, w488) -> (w491:cluster{dbl[], dbl[]})  [unwired: 1 in]
            n207 = Bundle(w489, w487) -> (w492:cluster{dbl[], dbl[]})  [unwired: 1 in]
            n208 = Bundle(w489, w486) -> (w493:cluster{dbl[], dbl[]})  [unwired: 1 in]
            n209 = Bundle(w489, w485) -> (w494:cluster{dbl[], dbl[]})  [unwired: 1 in]
            n210 = Bundle(w489, w484) -> (w495:cluster{dbl[], dbl[]})  [unwired: 1 in]
            n211 = Bundle(w489, w483) -> (w496:cluster{dbl[], dbl[]})  [unwired: 1 in]
            n212 = Bundle(w489, w482) -> (w497:cluster{dbl[], dbl[]})  [unwired: 1 in]
            n213 = Build Array(w491, w492, w493, w494, w495, w496, w497) -> (w490:cluster{dbl[], dbl[]}[])
          }
          frame "V, Lock-In X" {
            n214 = property on="MULTIPLE GRAPHS" class="XYGraph (strict)"("XScale.NameLbl.Text"="Lock-In X, V" ("X Scale.Name Label.Text")) -> ()  [unwired: 2 in, 2 out]
            n215 = Bundle(w506, w505) -> (w508:cluster{dbl[], dbl[]})  [unwired: 1 in]
            n216 = Bundle(w506, w504) -> (w509:cluster{dbl[], dbl[]})  [unwired: 1 in]
            n217 = Bundle(w506, w503) -> (w510:cluster{dbl[], dbl[]})  [unwired: 1 in]
            n218 = Bundle(w506, w502) -> (w511:cluster{dbl[], dbl[]})  [unwired: 1 in]
            n219 = Bundle(w506, w501) -> (w512:cluster{dbl[], dbl[]})  [unwired: 1 in]
            n220 = Bundle(w506, w500) -> (w513:cluster{dbl[], dbl[]})  [unwired: 1 in]
            n221 = Bundle(w506, w499) -> (w514:cluster{dbl[], dbl[]})  [unwired: 1 in]
            n222 = Build Array(w508, w509, w510, w511, w512, w513, w514) -> (w507:cluster{dbl[], dbl[]}[])
          }
          frame "V, Lock-In Y" {
            n223 = property on="MULTIPLE GRAPHS" class="XYGraph (strict)"("XScale.NameLbl.Text"="Lock-In Y, V" ("X Scale.Name Label.Text")) -> ()  [unwired: 2 in, 2 out]
            n224 = Bundle(w523, w522) -> (w531:cluster{dbl[], dbl[]})  [unwired: 1 in]
            n225 = Bundle(w523, w521) -> (w530:cluster{dbl[], dbl[]})  [unwired: 1 in]
            n226 = Bundle(w523, w520) -> (w529:cluster{dbl[], dbl[]})  [unwired: 1 in]
            n227 = Bundle(w523, w519) -> (w528:cluster{dbl[], dbl[]})  [unwired: 1 in]
            n228 = Bundle(w523, w518) -> (w527:cluster{dbl[], dbl[]})  [unwired: 1 in]
            n229 = Bundle(w523, w517) -> (w526:cluster{dbl[], dbl[]})  [unwired: 1 in]
            n230 = Bundle(w523, w516) -> (w525:cluster{dbl[], dbl[]})  [unwired: 1 in]
            n231 = Build Array(w531, w530, w529, w528, w527, w526, w525) -> (w524:cluster{dbl[], dbl[]}[])
          }
        }
        "MULTIPLE GRAPHS" <- w205
        n232 = Unbundle(w214) -> (w241:dbl[], w240:dbl[], w239:dbl[], w238:dbl[], w237:dbl[], w236:dbl[], w235:dbl[], w234:dbl[], w233:dbl[])
        "2000" <- w376
        "DAQ A0" <- w186
        "DAQ A1" <- w185
        "DAQ A2" <- w184
        "DAQ A3" <- w183
        "DAQ A4" <- w187
      }
    }
    frame #3 {
      # "Closing instrumental \nconnections"
      n233 = Unbundle(w749) -> ("Task out"=w748:i32, "error out"=w747:errorcluster)
      n234 = call <instrlib>:"Close.vi"("VISA resource name"=w754, "error in (no error)"=w755) -> ()  [unwired: 17 in, 1 out]
      n235 = call "SR51XX Close"("error in (no error)"=w750, "VISA session"=w751) -> ()  [unwired: 1 out]
      n236 = call <instrlib>:"Close.vi"("VISA resource name"=w752, "error in (no error)"=w753) -> ()  [unwired: 13 in, 1 out]
      n237 = call <userlib>:"DtOLCloseTask.vi"("Error in"=w747, "Task in"=w748) -> ("Error Out"=w756:errorcluster)  [unwired: 9 in]
      n238 = call <vilib>:"Simple Error Handler.vi"("error in (no error)"=w756) -> ()  [unwired: 4 in, 5 out]
    }
  }
